vi "PI-sctl-3.vi"(6 "Ready For Output":bool, 8 "Input Valid":bool, 9 "phase error":fxp<+/-,16,2>, 10 "param":T1={"base freq (Hz)"=[20123.0, 20123.0, 20123.0], "P gain"=[1234.0, 1234.0, 1234.0], "I gain"=[1.0, 1.0, 1.0], "LP1 coeffs"=[-1025014616, 2098093632, 165702, -1053286467, 2126356551, 167935, -1025014616, 2098093632, 165702, -1053286467, 2126356551, 167935, -1025014616, 2098093632, 165702, -1053286467, 2126356551, 167935], "scope on"=FALSE, "scope channel"=0, "scope signal"=0, "notch coeff"=[-1025014616, 2098093632, 165702, -1053286467, 2126356551, 167935, -1025014616, 2098093632, 165702]}, 11 "reset":bool) -> (0 "Output Valid":bool, 1 "freq. error":fxp<+/-,19,11> format="%.14g", 2 "freq error mean out":fxp<+/-,16,11>[](array[numeric]), 3 "phase errror mean out":fxp<+,16,1>[](array[numeric]), 4 "Ready For Input":bool=TRUE, 5 "freq errors out":fxp<+/-,16,1>[](array[numeric]), 7 "phase errrors out":fxp<+/-,16,1>[](array[numeric]))   [LabVIEW 2018, in "SCTL.lvlib"]
doc: "This VI is used in four wire handshake."
uses:
  SCTL.lvlib
  param-sctl-pll.ctl
  <vilib>/rvi/FXPMathLib/basic elements/FxpIntAccumulator/subVIs/nifxpmath_IntAccumulator_SimConfig.ctl
  <vilib>/rvi/FXPMathLib/basic elements/FxpIntAccumulator/simVIs/DllFxpIntAccumulator_sub.vi
  <vilib>/rvi/FXPMathLib/FxpInterpret/XNode/nifxpmath_Interpret.xnode
  <vilib>/rvi/FXPMathLib/FxpAdd/XNode/nifxpmath_Add.xnode
  <vilib>/rvi/FXPMathLib/FxpMul/XNode/nifxpmath_Multiplier.xnode
  <vilib>/rvi/FXPMathLib/basic elements/FxpIntAccumulator/XNode/nifxpmath_IntAccumulator.xnode
  <vilib>/rvi/FXPMathLib/sim/FxpSim.dll
panel:
  # "Inputs"
  # "Outputs"
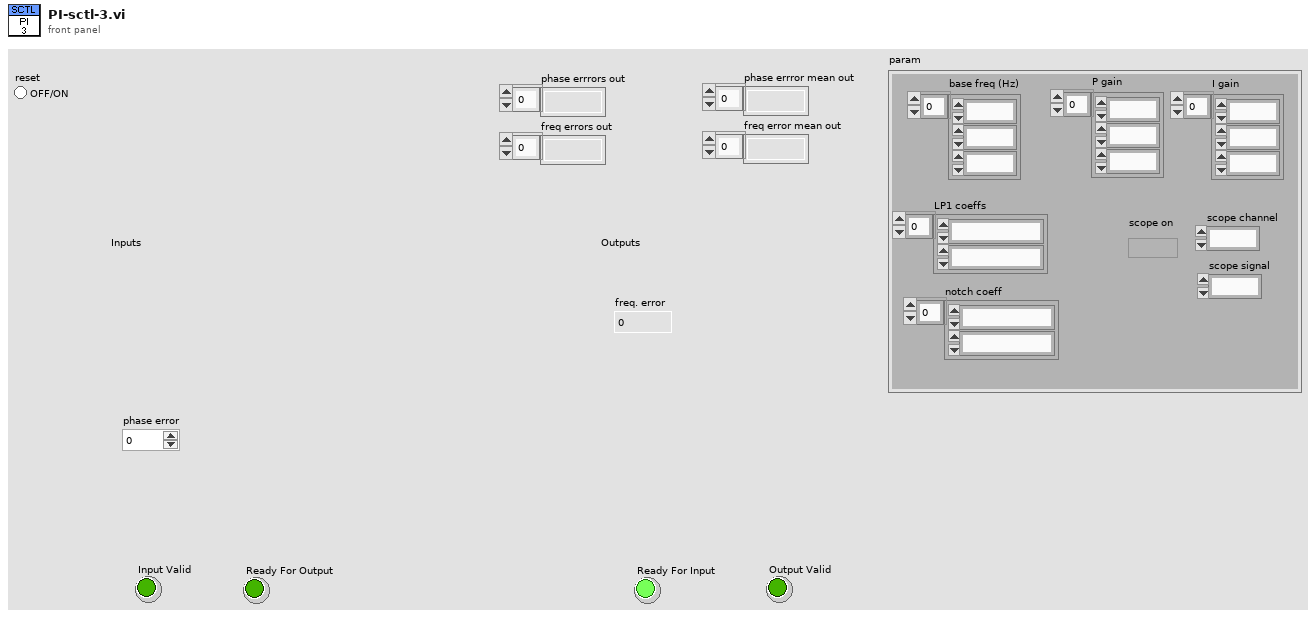
[diagram p1: front panel]
types:
  T1 = typedef "SCTL.lvlib/param-sctl-pll.ctl" = cluster{"base freq (Hz)":fxp<+,17,17>[], "P gain":fxp<+,14,14>[], "I gain":fxp<+,20,6>[], "LP1 coeffs":i32[], "scope on":bool, "scope channel":u8, "scope signal":u8, "notch coeff":i32[]}
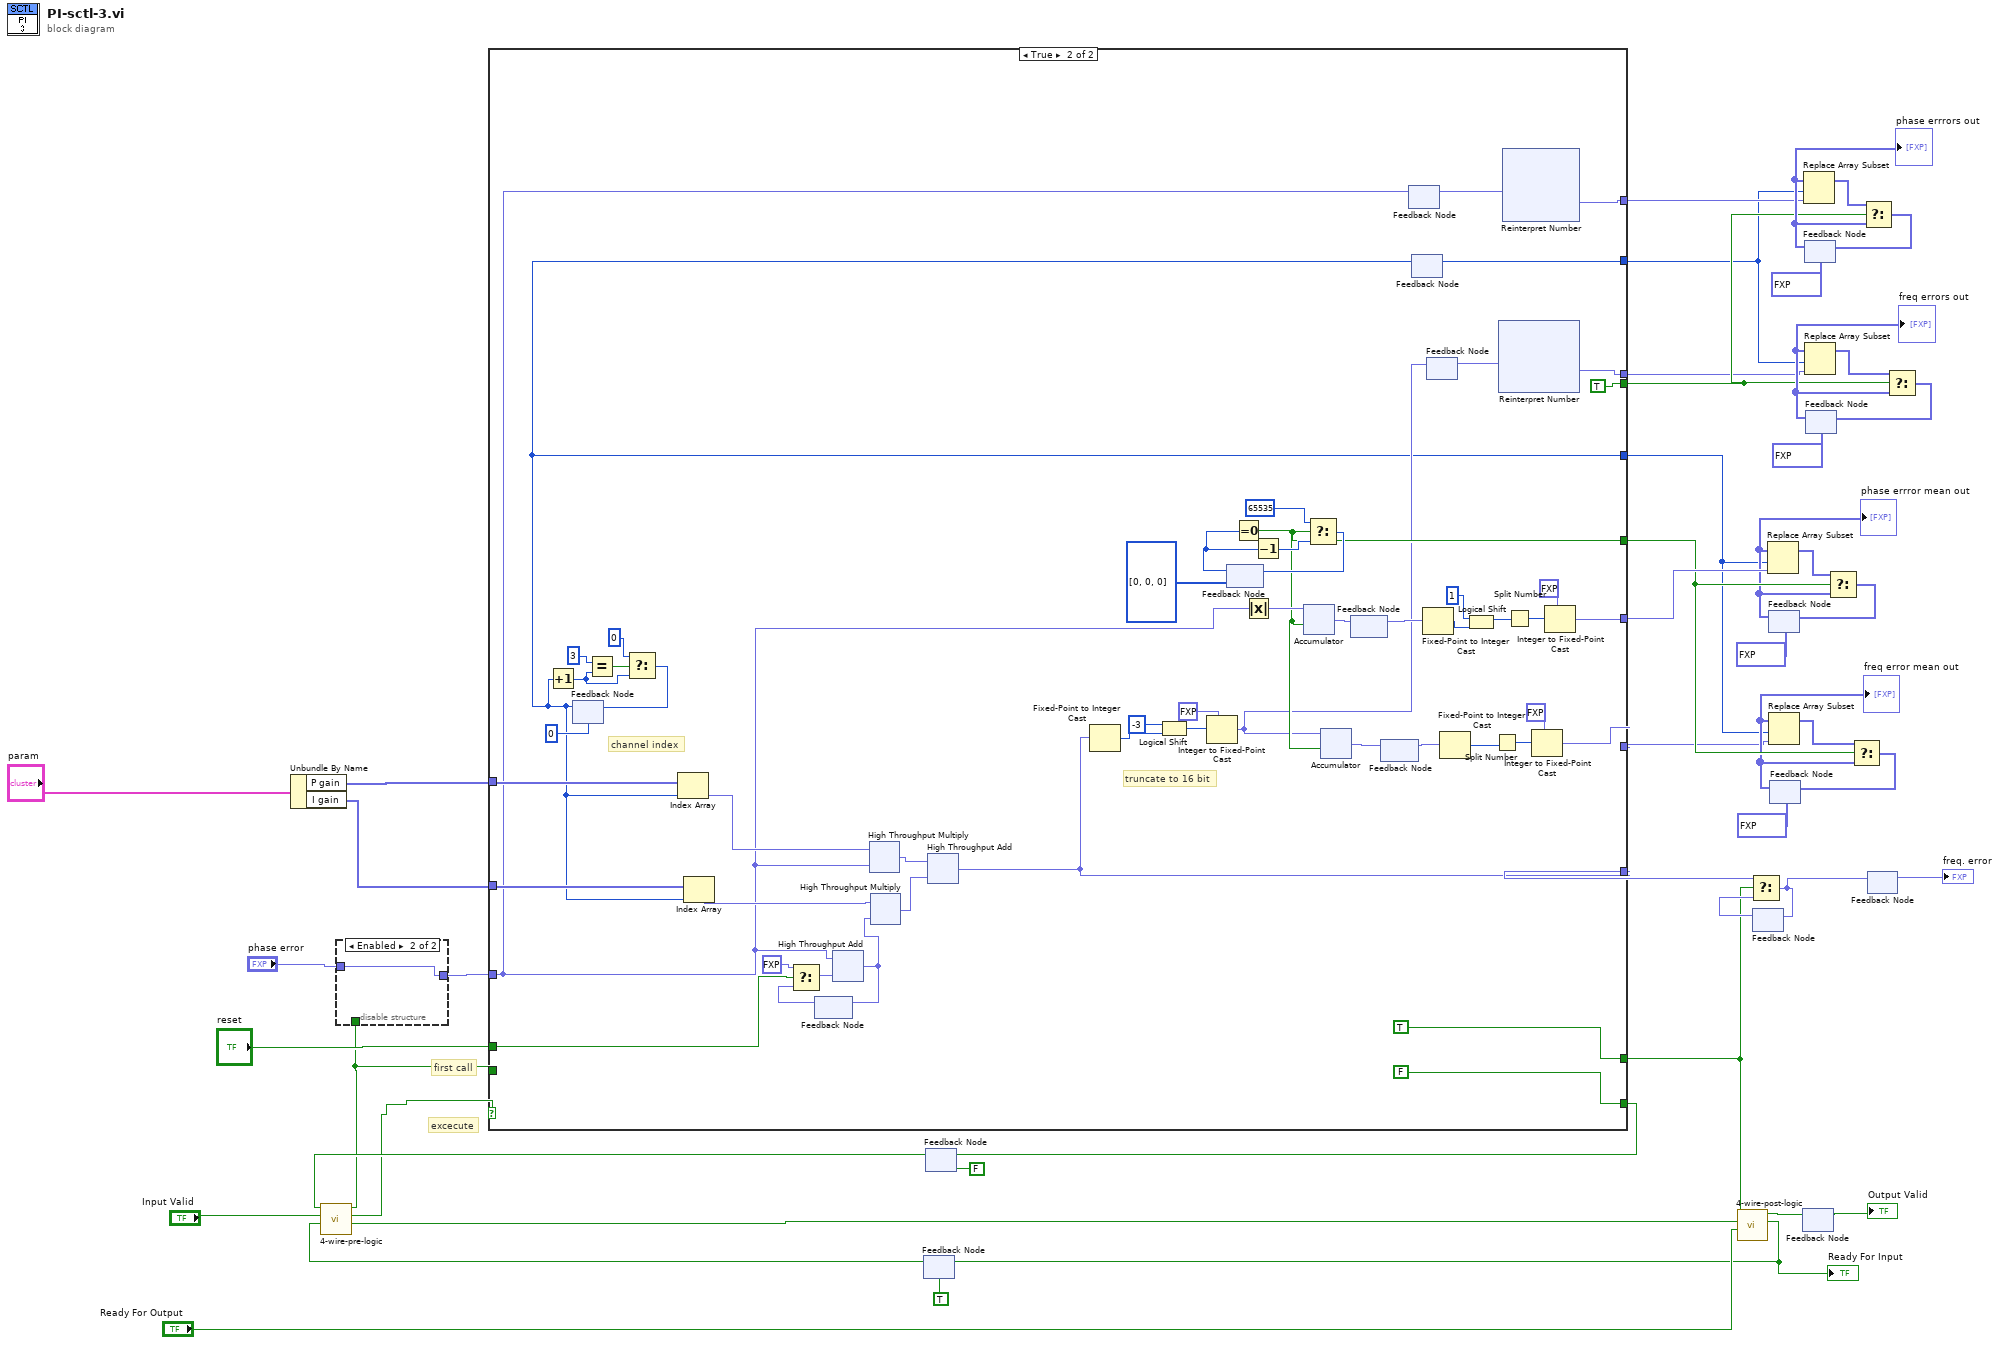
[diagram p0: block diagram]
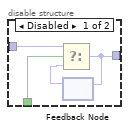
[diagram p2: hidden frame]
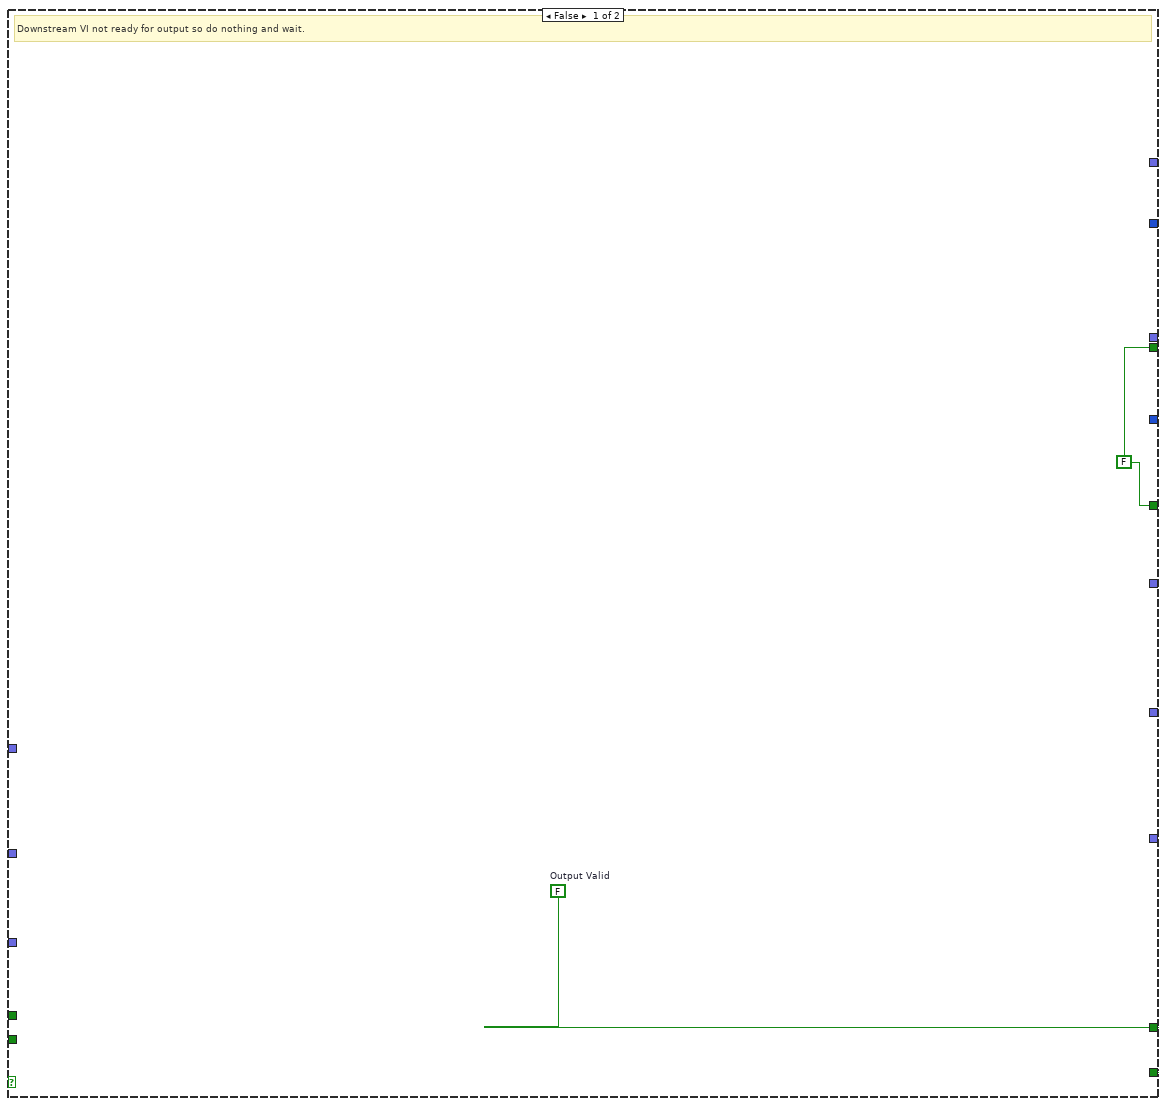
[diagram p3: hidden frame]
diagram:
  # "excecute"
  # "first call"
  n1 = Unbundle By Name("param") -> ("P gain"=w17:fxp<+,14,14>[], "I gain"=w16:fxp<+,20,6>[])
  n2 = feedback #1(TRUE ("x .and. y?")) -> (w43:bool)
  n3 = feedback #2(FALSE ("x .and. y?")) -> (w41:bool)
  n4 = call "4-wire-pre-logic.vi"("ready for input in"=w43, "Input Valid in"="Input Valid", "needs more iter in"=w41) -> ("register state out"=w47:bool, "excecute"=w31:bool, "buffer input!"=w32:bool)  [unwired: 6 in]
  n5 = disable-structure shown="Enabled" {
    disable-tunnel: "phase error" -> [w51 w53]
    disable-tunnel: [w50 w53] -> w35
    disable-tunnel: w32 -> [w49 _]
    frame Disabled {
      n6 = feedback #3() -> (w52:fxp<+/-,16,2>)  [unwired: 1 in]
      n7 = Select(t=w51, s=w49, f=w52) -> (s? t:f=w50:fxp<+/-,16,2>)
      n8 = feedback-in #3(w50) -> ()
    }
    frame Enabled {
    }
  }
  n9 = case shown="True" w31 {
    tunnel: [w55 TRUE ("Output Valid")] -> w45
    tunnel: w32 -> [_ _]
    tunnel: [w55 FALSE] -> w40
    tunnel: w35 -> [_ w63]
    tunnel: "reset" -> [_ w104]
    tunnel: [_ w64] -> w33
    tunnel: [w54 w66] -> w20
    tunnel: [_ w81] -> w25
    tunnel: [_ w57] -> w5
    tunnel: [_ w71] -> w14
    tunnel: w17 -> [_ w70]
    tunnel: w16 -> [_ w69]
    tunnel: [w54 TRUE ("x = 0?")] -> w4
    tunnel: [_ w62] -> w3
    tunnel: [_ w60] -> w2
    tunnel: [_ w56] -> w1
    frame False {
      w54 = FALSE
      w55 = FALSE  # Output Valid
      # "Downstream VI not ready for output so do nothing and wait."
    }
    frame True {
      # "truncate to 16 bit"
      # "channel index"
      n10 = feedback #4(i16 0) -> (w57:i16)
      n11 = Increment(x=w57) -> (x+1=w95:i16)
      n12 = Equal?(x=i16 3, y=w95) -> (x = y?=w100:bool)
      n13 = Select(t=i16 0, s=w100, f=w95) -> (s? t:f=w97:i16)
      n14 = feedback-in #4(w97) -> ()
      n15 = Index Array(array=w70, index=w57) -> (element=w68:fxp<+,14,14>)
      n16 = Index Array(array=w69, index=w57) -> (element=w67:fxp<+,20,6>)
      n17 = feedback #5() -> (w107:fxp<+/-,21,11>)  [unwired: 1 in]
      n18 = Select(t=fxp<+/-,21,10> 0.0, s=w104, f=w107) -> (s? t:f=w105:fxp<+/-,22,11>)
      n19 = xnode ("High Throughput Add")("x"=w63, "y"=w105) -> ("x+y"=w103:fxp<+/-,21,11>)
      n20 = feedback-in #5(w103) -> ()
      n21 = xnode ("High Throughput Multiply")("x"=w68, "y"=w63) -> ("x*y"=w108:fxp<+/-,19,11>)
      n22 = xnode ("High Throughput Multiply")("x"=w67, "y"=w103) -> ("x*y"=w109:fxp<+/-,19,11>)
      n23 = xnode ("High Throughput Add")("x"=w108, "y"=w109) -> ("x+y"=w64:fxp<+/-,19,11>)
      n24 = Fixed-Point to Integer Cast(1:w64) -> (0:w75:i32)
      n25 = Logical Shift(y=i16 -3, x=w75) -> (x << y=w74:i32)
      n26 = Integer to Fixed-Point Cast(fixed-point type=fxp<+/-,16,11> 0.0 ("fixed-point"), integer=w74) -> (fixed-point=w61:fxp<+/-,16,11>)
      n27 = feedback #6(u16[] [0, 0, 0]) -> (w83:u16)
      n28 = Equal To 0?(x=w83) -> (x = 0?=w66:bool)
      n29 = Absolute Value(x=w63) -> (abs(x)=w93:fxp<+,16,2>)
      n30 = Decrement(x=w83) -> (x-1=w87:u16)
      n31 = xnode "Accumulator"("x"=w93, "load (F)"=w66) -> ("s"=w86:fxp<+,32,18>)  [unwired: 3 in, 1 out]
      n32 = Select(t=u16 65535, s=w66, f=w87) -> (s? t:f=w94:u16)
      n33 = feedback-in #6(w94) -> ()
      n34 = xnode "Accumulator"("x"=w61, "load (F)"=w66) -> ("s"=w78:fxp<+/-,32,27>)  [unwired: 3 in, 1 out]
      n35 = feedback #7() -> (w85:fxp<+,32,18>)  [unwired: 1 in]
      n36 = feedback-in #7(w86) -> ()
      n37 = feedback #8() -> (w77:fxp<+/-,32,27>)  [unwired: 1 in]
      n38 = feedback-in #8(w78) -> ()
      n39 = feedback-in #9(w63) -> ()
      n40 = feedback #9() -> (w58:fxp<+/-,16,2>)  [unwired: 1 in]
      n41 = feedback-in #10(w57) -> ()
      n42 = feedback #10() -> (w56:i16)  [unwired: 1 in]
      n43 = Fixed-Point to Integer Cast(1:w85) -> (0:w90:u32)
      n44 = feedback-in #11(w61) -> ()
      n45 = feedback #11() -> (w59:fxp<+/-,16,11>)  [unwired: 1 in]
      n46 = Fixed-Point to Integer Cast(1:w77) -> (0:w72:i32)
      n47 = Logical Shift(y=i16 1, x=w90) -> (x << y=w89:u32)
      n48 = Split Number(x=w72) -> (hi(x)=w79:u16)  [unwired: 1 out]
      n49 = xnode "Reinterpret Number"("x"=w59) -> ("y"=w60:fxp<+/-,16,1>)
      n50 = xnode "Reinterpret Number"("x"=w58) -> ("y"=w62:fxp<+/-,16,1>)
      n51 = Split Number(x=w89) -> (hi(x)=w91:u16)  [unwired: 1 out]
      n52 = Integer to Fixed-Point Cast(fixed-point type=fxp<+/-,16,11> 0.0 ("fixed-point"), integer=w79) -> (fixed-point=w71:fxp<+/-,16,11>)
      n53 = Integer to Fixed-Point Cast(fixed-point type=fxp<+,16,1> 0.0 ("fixed-point"), integer=w91) -> (fixed-point=w81:fxp<+,16,1>)
    }
  }
  n54 = feedback-in #2(w40) -> ()
  n55 = call "4-wire-post-logic.vi"("Ready For Output in"="Ready For Output", "register state in"=w47, "output valid in"=w45) -> ("ready for input out"=w37:bool, "output valid out"=w29:bool)  [unwired: 7 in]
  "Ready For Input" <- w37
  n56 = feedback-in #1(w37) -> ()
  n57 = feedback #12() -> (w46:fxp<+/-,19,11>)  [unwired: 1 in]
  n58 = Select(t=w33, s=w45, f=w46) -> (s? t:f=w44:fxp<+/-,19,11>)
  n59 = feedback-in #12(w44) -> ()
  n60 = feedback #13(fxp<+,16,1>[] [0.0, 0.0, 0.0] ("s? t:f")) -> (w19:fxp<+,16,1>[])
  "phase errror mean out" <- w19
  n61 = Replace Array Subset(array=w19, new element=w25, index=w5) -> (w27:fxp<+,16,1>[])
  n62 = feedback #14(fxp<+/-,16,11>[] [0.0, 0.0, 0.0] ("s? t:f")) -> (w18:fxp<+/-,16,11>[])
  "freq error mean out" <- w18
  n63 = Replace Array Subset(array=w18, new element=w14, index=w5) -> (w23:fxp<+/-,16,11>[])
  n64 = feedback #15() -> (→"Output Valid":bool)  [unwired: 1 in]
  n65 = feedback-in #15(w29) -> ()
  n66 = feedback #16(fxp<+/-,16,1>[] [0.0, 0.0, 0.0] ("s? t:f")) -> (w7:fxp<+/-,16,1>[])
  "phase errrors out" <- w7
  n67 = Replace Array Subset(array=w7, new element=w3, index=w1) -> (w13:fxp<+/-,16,1>[])
  n68 = feedback #17(fxp<+/-,16,1>[] [0.0, 0.0, 0.0] ("s? t:f")) -> (w6:fxp<+/-,16,1>[])
  "freq errors out" <- w6
  n69 = Replace Array Subset(array=w6, new element=w2, index=w1) -> (w10:fxp<+/-,16,1>[])
  n70 = Select(t=w27, s=w20, f=w19) -> (s? t:f=w24:fxp<+,16,1>[])
  n71 = feedback-in #13(w24) -> ()
  n72 = Select(t=w23, s=w20, f=w18) -> (s? t:f=w21:fxp<+/-,16,11>[])
  n73 = feedback-in #14(w21) -> ()
  n74 = Select(t=w13, s=w4, f=w7) -> (s? t:f=w11:fxp<+/-,16,1>[])
  n75 = feedback-in #16(w11) -> ()
  n76 = feedback-in #18(w44) -> ()
  n77 = feedback #18() -> (→"freq. error":fxp<+/-,19,11>)  [unwired: 1 in]
  n78 = Select(t=w10, s=w4, f=w6) -> (s? t:f=w8:fxp<+/-,16,1>[])
  n79 = feedback-in #17(w8) -> ()
